vi "Queue Msg To Nested.vi"(8 "Alias":string, 9 "Priority?":bool, 10 "Msg":refnum<class "Msg.lvclass">, 11 "jettl Queue Actor in":refnum<class "jettl Queue Actor.lvclass">) -> (0 "error out":errorcluster)   [LabVIEW 2021, in "jettl.lvlib" / "jettl Queue Actor.lvlib" / "jettl Queue Actor.lvclass"]
uses:
  jettl Queue Actor.lvclass
  Actor/Msg/Msg.lvclass
  jettl Queue Actor.lvclass/jettl Queue Actor.ctl
  jettl.lvlib
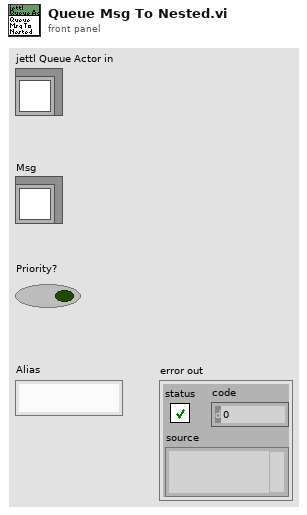
[diagram p1: front panel]
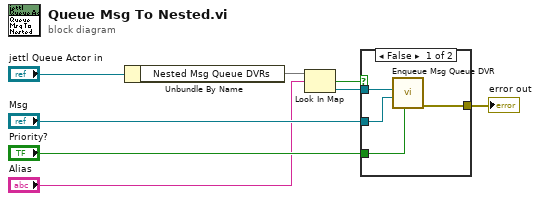
[diagram p0: block diagram]
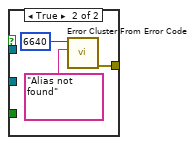
[diagram p2: hidden frame]
diagram:
  n1 = Unbundle By Name("jettl Queue Actor in") -> ("Nested Msg Queue DVRs"=w4:map{string, refnum<data-value>})
  n2 = Look In Map(map=w4, key="Alias") -> (key not found?=w1:bool, value=w3:refnum<data-value>)  [unwired: 1 in]
  n3 = case shown="False" w1 {
    tunnel: [w12 w15] -> w7
    tunnel: "Priority?" -> [w11 _]
    tunnel: "Msg" -> [w10 _]
    tunnel: w3 -> [w9 _]
    frame False {
      n4 = call "Enqueue Msg Queue DVR.vi"("Priority?"=w11, "Msg"=w10, "Msg Queue DVR"=w9) -> ("error out"=w12:errorcluster)  [unwired: 8 in]
    }
    frame True {
      n5 = call <vilib>:"Error Cluster From Error Code.vi"("error message (\"\")"="Alias not found" ("error message (\"\")"), "error code (0)"=6640) -> ("error out"=w15:errorcluster)  [unwired: 7 in]
    }
  }
  "error out" <- w7
